vi "PIDController_AtSetpoint.vi"(11 "in PID_CONTROLLER":T1={"Kp"=0.0, "Ki"=0.0, "Kd"=0.0, "Period"=0.0, "Max_Integral"=0.0, "Min_Integral"=0.0, "Max_Input"=0.0, "Min_Input"=0.0, "Continuous"=FALSE, "PositionError"=0.0, "VelocityError"=0.0, "PrevError"=0.0, "TotalError"=0.0, "PositionTolerance"=0.0, "VelocityTolerance"=0.0, "SetPoint"=0.0, "Kf"=0.0, "Prev_Deriv"=0.0, "Prev_Deriv 2"=0.0, "DerivativeFilter"=FALSE, "Min_Output"=-9.99e+35, "Max_Output"=9.9e+35, "Prev_F_P"=0.0, "Prev_F_P_2"=0.0, "AntiWindupActive"=FALSE, "Measurement"=0.0} {"Measurement" format="%16_6e"; "Prev_F_P_2" format="%16_6e"; "Prev_F_P" format="%16_6e"; "Max_Output" format="%16_6e"; "Min_Output" format="%16_6e"; "Prev_Deriv 2" format="%16_6e"; "Prev_Deriv" format="%16_6e"; "Kf" format="%16_6e"; "SetPoint" format="%16_6e"; "VelocityTolerance" format="%16_6e"; "PositionTolerance" format="%16_6e"; "TotalError" format="%16_6e"; "PrevError" format="%16_6e"; "VelocityError" format="%16_6e"; "PositionError" format="%16_6e"; "Min_Input" format="%16_6e"; "Max_Input" format="%16_6e"; "Min_Integral" format="%16_6e"; "Max_Integral" format="%16_6e"; "Period" format="%16_6e"; "Kd" format="%16_6e"; "Ki" format="%16_6e"; "Kp" format="%16_6e"}) -> (3 "AtSetpoint":bool)   [LabVIEW 2019, in "Trajectory_Library.lvlib"]
doc: "Returns true if the error is within the percentage of the total input range, determined by SetTolerance. This asssumes that the maximum and minimum input were set using SetInput.\n \nThis will return false until at least one input value has been computed.\n \nInputs:\n - PID_Controller -- PID_Controller data cluster\n\nOutputs:\n - AtSetpoint -- Whether the error is within the acceptable bounds."
uses:
  Trajectory_Library.lvlib
  PID_CONTROLLER.ctl
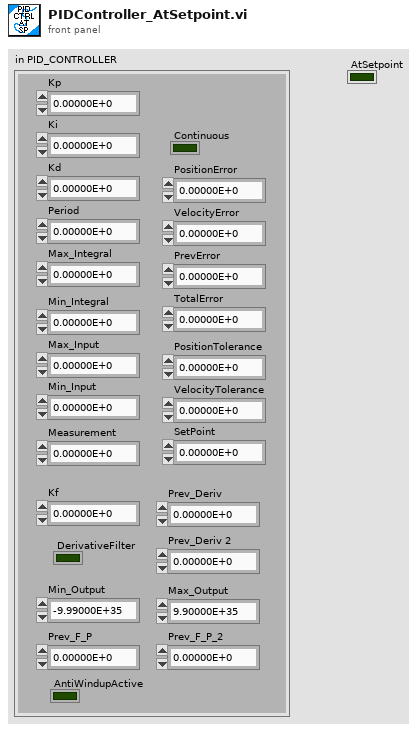
[diagram p1: front panel]
types:
  T1 = typedef "Trajectory_Library.lvlib/PID_CONTROLLER.ctl" = cluster{"Kp":dbl, "Ki":dbl, "Kd":dbl, "Period":dbl, "Max_Integral":dbl, "Min_Integral":dbl, "Max_Input":dbl, "Min_Input":dbl, "Continuous":bool, "PositionError":dbl, "VelocityError":dbl, "PrevError":dbl, "TotalError":dbl, "PositionTolerance":dbl, "VelocityTolerance":dbl, "SetPoint":dbl, "Kf":dbl, "Prev_Deriv":dbl, "Prev_Deriv 2":dbl, "DerivativeFilter":bool, "Min_Output":dbl, "Max_Output":dbl, "Prev_F_P":dbl, "Prev_F_P_2":dbl, "AntiWindupActive":bool, "Measurement":dbl}
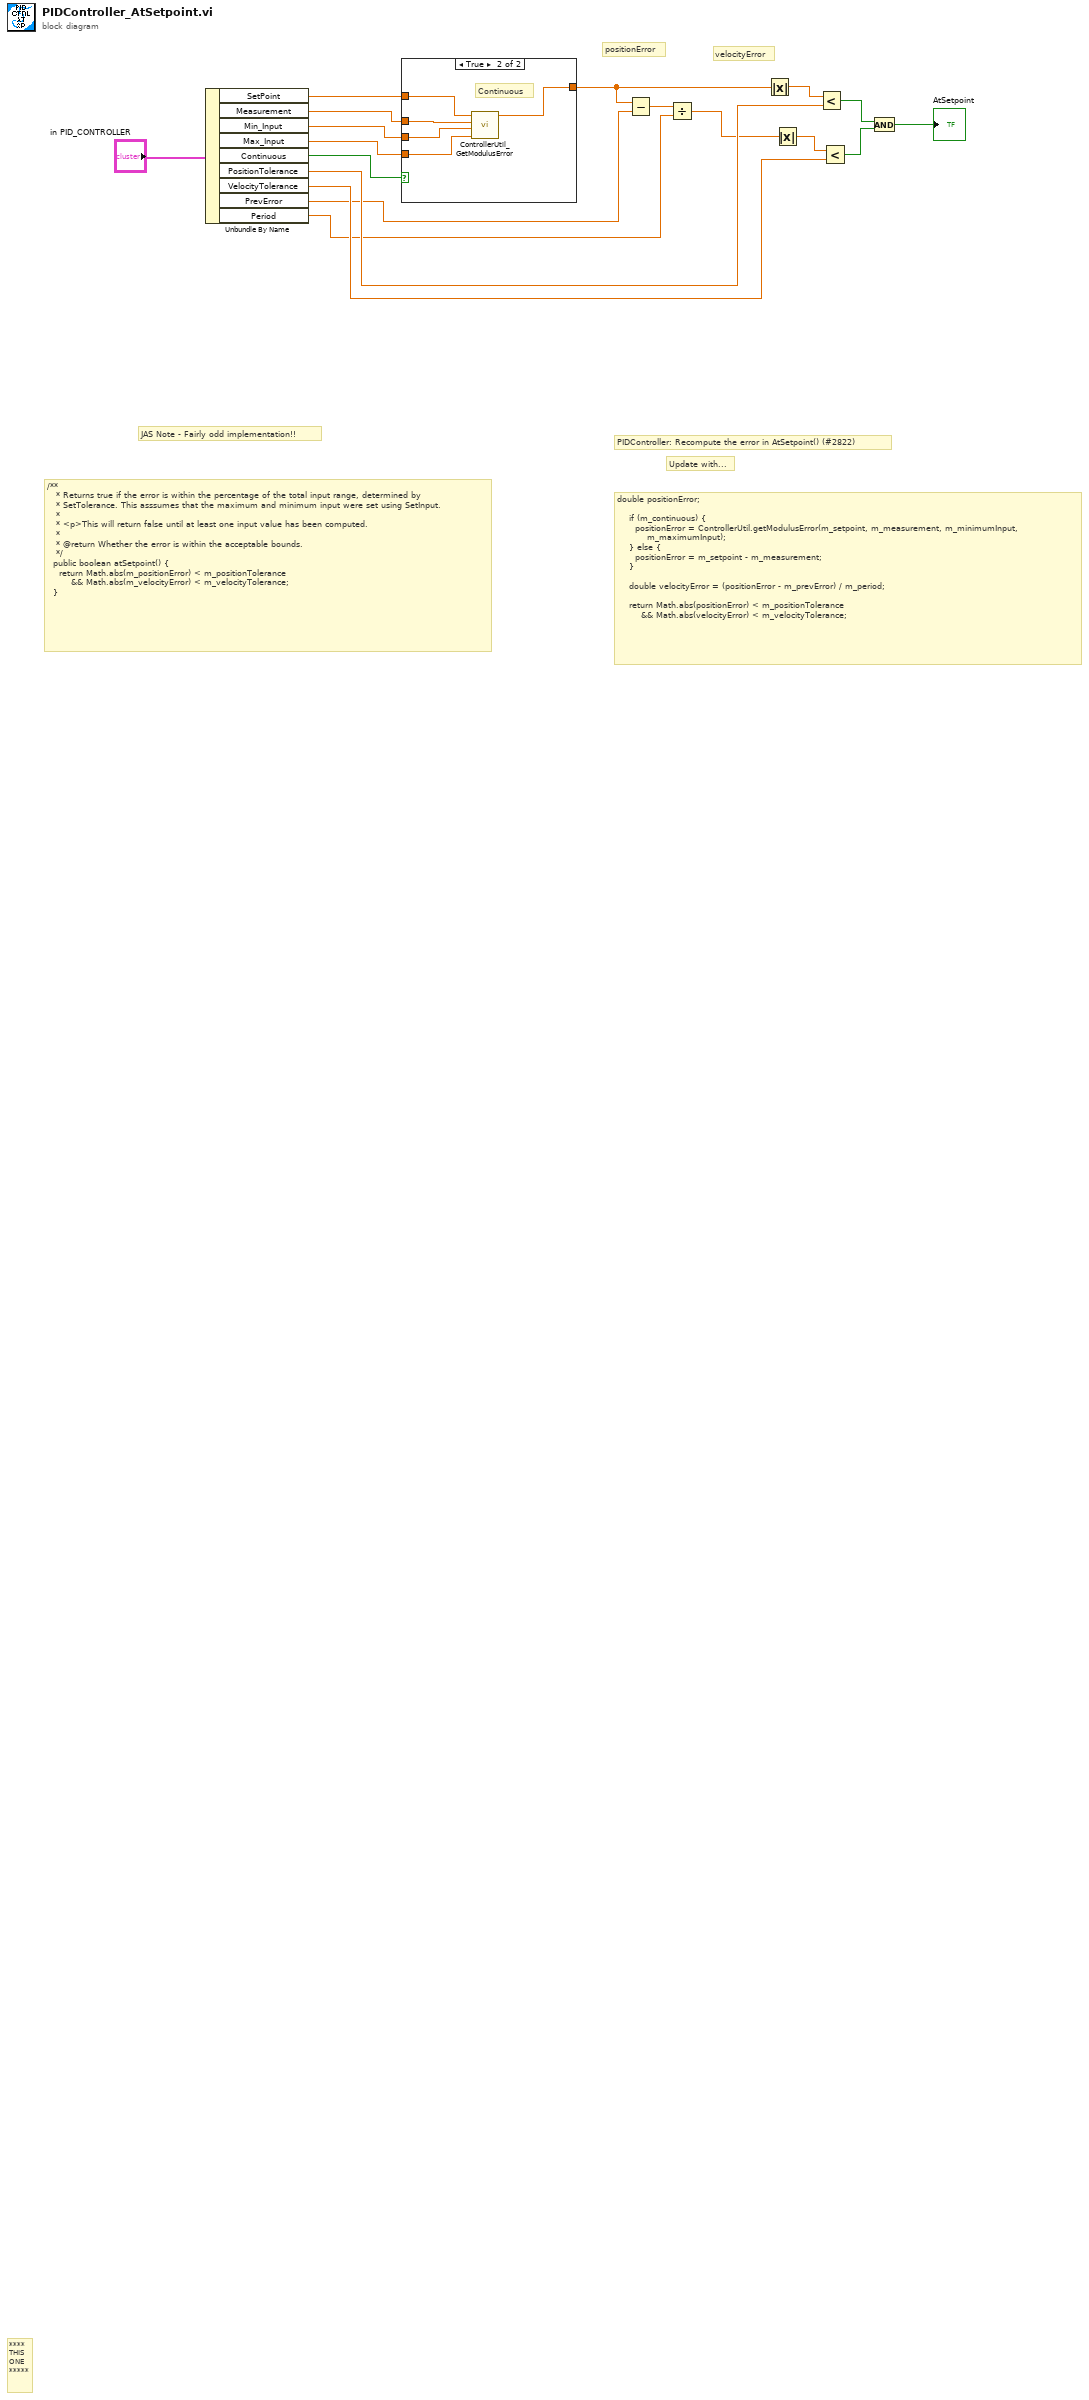
[diagram p0: block diagram]
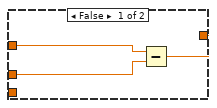
[diagram p2: hidden frame]
diagram:
  # "velocityError"
  # "positionError"
  # "Update with..."
  # "double positionError;\n\n    if (m_continuous) {\n      positionError = ControllerUtil.getModulusError(m_setpoint, m_measurement, m_minimumInput,\n          m_maximumInput);\n    } else {\n      positionError = m_setpoint - m_measurement;\n    }\n\n    double velocityError = (positionError - m_prevError) / m_period;\n\n    return Math.abs(positionError) < m_positionTolerance\n        && Math.abs(velocityError) < m_velocityTolerance;"
  # "PIDController: Recompute the error in AtSetpoint() (#2822)"
  # "JAS Note - Fairly odd implementation!!"
  # "/**\n   * Returns true if the error is within the percentage of the total input range, determined by\n   * SetTolerance. This asssumes that the maximum and minimum input were set using SetInput.\n   *\n   * <p>This will return false until at least one input value has been computed.\n   *\n   * @return Whether the error is within the acceptable bounds.\n   */\n  public boolean atSetpoint() {\n    return Math.abs(m_positionError) < m_positionTolerance\n        && Math.abs(m_velocityError) < m_velocityTolerance;\n  }"
  # "****\nTHIS\nONE\n*****"
  n1 = Unbundle By Name("in PID_CONTROLLER") -> ("SetPoint"=w11:dbl, "Measurement"=w10:dbl, "Min_Input"=w7:dbl, "Max_Input"=w6:dbl, "Continuous"=w12:bool, "PositionTolerance"=w9:dbl, "VelocityTolerance"=w8:dbl, "PrevError"=w4:dbl, "Period"=w2:dbl)
  n2 = case shown="True" w12 {
    tunnel: w11 -> [w21 w26]
    tunnel: w10 -> [w20 w25]
    tunnel: [w19 w22] -> w5
    tunnel: w7 -> [_ w24]
    tunnel: w6 -> [_ w23]
    frame False {
      n3 = Subtract(x=w21, y=w20) -> (x-y=w19:dbl)
    }
    frame True {
      # "Continuous"
      n4 = call "ControllerUtil_GetModulusError.vi"("Maximum_Input"=w23, "Minimum_Input"=w24, "Measurerment(PV)"=w25, "Reference(SP)"=w26) -> ("Error"=w22:dbl)  [unwired: 7 in]
    }
  }
  n5 = Subtract(x=w5, y=w4) -> (x-y=w3:dbl)
  n6 = Divide(x=w3, y=w2) -> (x/y=w1:dbl)
  n7 = Absolute Value(x=w5) -> (abs(x)=w17:dbl)
  n8 = Absolute Value(x=w1) -> (abs(x)=w16:dbl)
  n9 = Less?(x=w17, y=w9) -> (x < y?=w15:bool)
  n10 = Less?(x=w16, y=w8) -> (x < y?=w14:bool)
  n11 = And(x=w15, y=w14) -> (x .and. y?=→"AtSetpoint":bool)
